vi "add.vi"(8 "error in":errorcluster, 9 "value":string, 10 "name":string, 11 "properties in":refnum<class "properties.lvclass">) -> (0 "error out":errorcluster, 3 "properties out":refnum<class "properties.lvclass">)   [LabVIEW 2020, in "nominal types.lvlib" / "properties.lvclass"]
uses:
  properties.lvclass
  properties.lvclass/properties.ctl
  <vilib>/Utility/miscctls.llb/LVMapReplaceAction.ctl
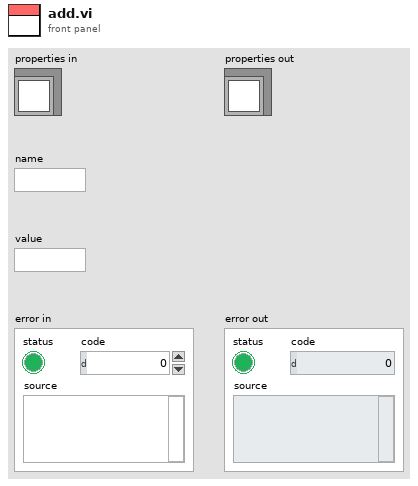
[diagram p1: front panel]
types:
  T1 = typedef "LVMapReplaceAction.ctl" = enum32{"Modify Entry only if found", "Add or Modify Entry", "Delete Entry"}
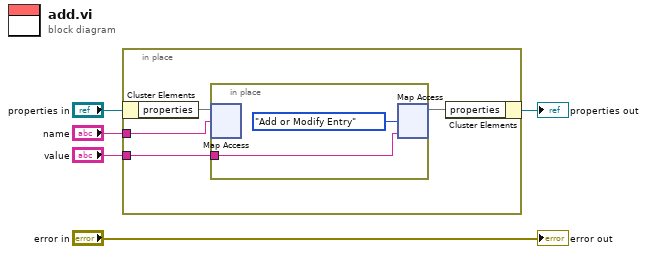
[diagram p0: block diagram]
diagram:
  n1 = in-place {
    in-place-border: "name" -> [w8]
    in-place-border: "value" -> [w7]
    n2 = in-place-cluster #1("properties in") -> ("properties"=w9:map{string, string})
    n3 = in-place {
      in-place-border: w7 -> [w10]
      n4 = in-place-map #2(w9, w8) -> ()  [unwired: 1 in, 2 out]
      n5 = in-place-map #2(w10, LVMapReplaceAction."Add or Modify Entry" ("action")) -> (w6:map{string, string})  [unwired: 2 out]
    }
    n6 = in-place-cluster #1("properties"=w6) -> (→"properties out":refnum<class "properties.lvclass">)
  }
  "error out" <- "error in"
